vi "limelight-turret_converter.vi"(0 "Psi":dbl, 1 "Delta":dbl, 2 "Radius":dbl) -> ()   [LabVIEW 2019]
panel:
  out "D^2":dbl
  out "Theta":dbl
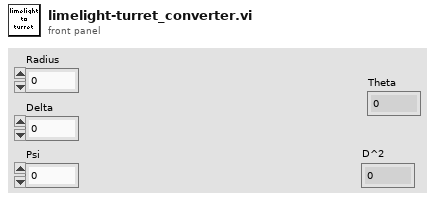
[diagram p1: front panel]
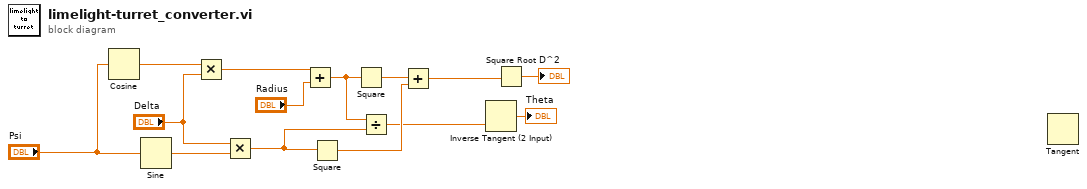
[diagram p0: block diagram]
diagram:
  n1 = Cosine(x="Psi") -> (cos(x)=w3:dbl)
  n2 = Sine(x="Psi") -> (sin(x)=w12:dbl)
  n3 = Multiply(x=w3, y="Delta") -> (x*y=w14:dbl)
  n4 = Multiply(x="Delta", y=w12) -> (x*y=w6:dbl)
  n5 = Add(x=w14, y="Radius") -> (x+y=w7:dbl)
  n6 = Square(x=w6) -> (x^2=w10:dbl)
  n7 = Square(x=w7) -> (x^2=w11:dbl)
  n8 = Divide(x=w7, y=w6) -> (x/y=w5:dbl)
  n9 = Add(x=w11, y=w10) -> (x+y=w9:dbl)
  n10 = Inverse Tangent (2 Input)(1:w5) -> (0:→"Theta":dbl)  [unwired: 1 in]
  n11 = Square Root(x=w9) -> (sqrt(x)=→"D^2":dbl)
  n12 = Tangent() -> ()  [unwired: 1 in, 1 out]
